vi "ES Randomize Infos.vi"(10 "DeviceID":T2) -> (3 "ES_Info Array out":T1[](array[typedef]))   [LabVIEW 2018, in "IED Test Framework.lvlib" / "IED Test.lvclass"]
uses:
  IED Test.lvclass
  <vilib>/ORNL/CSEISMIC DDS/CSEISMIC DDS Base/Data Types/Controls/DeviceID.ctl
  <vilib>/ORNL/CSEISMIC DDS/CSEISMIC DDS Base/Data Types/ES_Info.ctl
  <vilib>/ORNL/CSEISMIC DDS/CSEISMIC DDS Base/Data Types/Controls/EfficiencyCurve.ctl
  <vilib>/ORNL/CSEISMIC DDS/CSEISMIC DDS Base/CSEISMIC DDS.lvclass
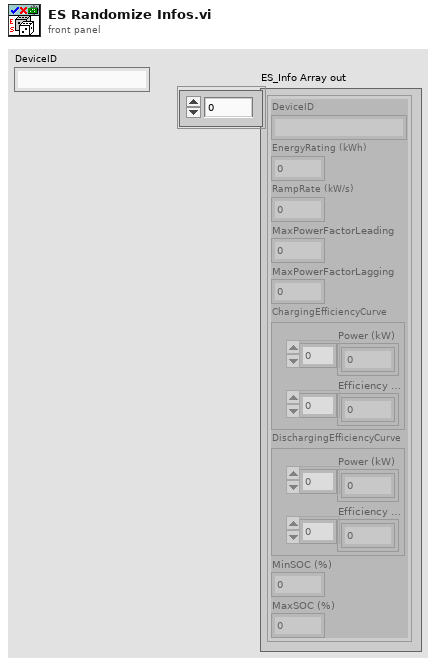
[diagram p1: front panel]
types:
  T1 = typedef "CSEISMIC DDS.lvlib/CSEISMIC DDS.lvclass/ES_Info.ctl" = cluster{"DeviceID":T2, "EnergyRating (kWh)":dbl, "RampRate (kW/s)":dbl, "MaxPowerFactorLeading":dbl, "MaxPowerFactorLagging":dbl, "ChargingEfficiencyCurve":T3, "DischargingEfficiencyCurve":T3, "MinSOC (%)":dbl, "MaxSOC (%)":dbl}
  T2 = typedef "CSEISMIC DDS.lvlib/CSEISMIC DDS.lvclass/DeviceID.ctl" = string
  T3 = typedef "CSEISMIC DDS.lvlib/CSEISMIC DDS.lvclass/EfficiencyCurve.ctl" = cluster{"Power (kW)":dbl[], "Efficiency (%)":dbl[]}
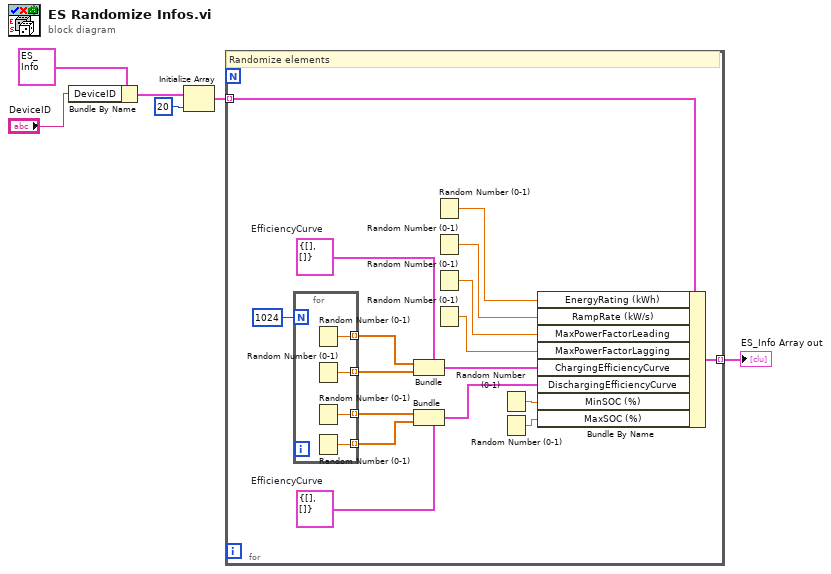
[diagram p0: block diagram]
diagram:
  n1 = Bundle By Name(cluster=T1 {"DeviceID"="", "EnergyRating (kWh)"=0.0, "RampRate (kW/s)"=0.0, "MaxPowerFactorLeading"=0.0, "MaxPowerFactorLagging"=0.0, "ChargingEfficiencyCurve"={"Power (kW)"=array[1024 elements], "Efficiency (%)"=array[1024 elements]}, "DischargingEfficiencyCurve"={"Power (kW)"=array[1024 elements], "Efficiency (%)"=array[1024 elements]}, "MinSOC (%)"=0.0, "MaxSOC (%)"=0.0} ("ES_Info"), "DeviceID"="DeviceID") -> (w5:T1)
  n2 = Initialize Array(w5, 20 ("dimension size")) -> (w2:T1[])
  n3 = for {
    tunnel: w2 -> [w23] mode=indexing
    tunnel: [w22] -> w1 mode=indexing
    w7 = T3 {"Power (kW)"=[], "Efficiency (%)"=[]}  # EfficiencyCurve
    w8 = T3 {"Power (kW)"=[], "Efficiency (%)"=[]}  # EfficiencyCurve
    # "Randomize elements"
    n4 = for {
      N: 1024 -> [_]
      tunnel: [w27] -> w16 mode=indexing
      tunnel: [w26] -> w15 mode=indexing
      tunnel: [w25] -> w13 mode=indexing
      tunnel: [w24] -> w12 mode=indexing
      n5 = Random Number (0-1)() -> (number: 0 to 1=w27:dbl)
      n6 = Random Number (0-1)() -> (number: 0 to 1=w26:dbl)
      n7 = Random Number (0-1)() -> (number: 0 to 1=w25:dbl)
      n8 = Random Number (0-1)() -> (number: 0 to 1=w24:dbl)
    }
    n9 = Bundle(cluster=w8, "Power (kW)"=w16, "Efficiency (%)"=w15) -> (w14:T3)
    n10 = Bundle(cluster=w7, "Power (kW)"=w13, "Efficiency (%)"=w12) -> (w11:T3)
    n11 = Random Number (0-1)() -> (number: 0 to 1=w21:dbl)
    n12 = Random Number (0-1)() -> (number: 0 to 1=w20:dbl)
    n13 = Random Number (0-1)() -> (number: 0 to 1=w19:dbl)
    n14 = Random Number (0-1)() -> (number: 0 to 1=w18:dbl)
    n15 = Random Number (0-1)() -> (number: 0 to 1=w10:dbl)
    n16 = Random Number (0-1)() -> (number: 0 to 1=w9:dbl)
    n17 = Bundle By Name(cluster=w23, "EnergyRating (kWh)"=w21, "RampRate (kW/s)"=w20, "MaxPowerFactorLeading"=w19, "MaxPowerFactorLagging"=w18, "ChargingEfficiencyCurve"=w14, "DischargingEfficiencyCurve"=w11, "MinSOC (%)"=w10, "MaxSOC (%)"=w9) -> (w22:T1)
  }
  "ES_Info Array out" <- w1
